vi "RTD_inverse_polynome.vi"(5 "t stop":dbl=95.0, 7 "t start":dbl=5.0, 8 "error in":errorcluster, 11 "channel in":T1={"type"=enum."COMET Tx5xx (ethernet)", "comment"="", "tag"="", "refresh"=5.0, "IP"="192.168.2.34", "port"=502, "VISA"="", "last readout"=timestamp(0 s since 1904-01-01), "TCP ref"=refnum, "VISA sess"="", "idn"="", "press"=0.0, "RH"=0.0, "temp"=0.0, "pres cor"=[], "RH cor"=[], "temp cor"=[], "try left"=0, "failed"=FALSE, "RTD set"=[], "RTD inv"=[], "range"=0.0, "net mode"=enum."MODBUS", "try fail"=enum."Stop trying - return NaN", "timeout [s]"=0.0, "max retries"=0, "sim t [deg]"=0.0, "status"=0} {"status" items=["ok", "retry", "failed"]; "RTD inv" format="%.1f"; "RTD set" format="%.1f"; "temp cor" format="%.1f"; "RH cor" format="%.1f"; "pres cor" format="%.1f"; "refresh" min=0.1 max=1000.0 format="%.2f"}) -> (0 "error out":errorcluster, 3 "channel out":T1={"type"=enum."COMET Tx5xx (ethernet)", "comment"="", "tag"="", "refresh"=5.0, "IP"="192.168.2.34", "port"=502, "VISA"="", "last readout"=timestamp(0 s since 1904-01-01), "TCP ref"=refnum, "VISA sess"="", "idn"="", "press"=0.0, "RH"=0.0, "temp"=0.0, "pres cor"=[], "RH cor"=[], "temp cor"=[], "try left"=0, "failed"=FALSE, "RTD set"=[], "RTD inv"=[], "range"=0.0, "net mode"=enum."MODBUS", "try fail"=enum."Stop trying - return NaN", "timeout [s]"=0.0, "max retries"=0, "sim t [deg]"=0.0, "status"=0} {"status" items=["ok", "retry", "failed"]; "RTD inv" format="%.1f"; "RTD set" format="%.1f"; "temp cor" format="%.1f"; "RH cor" format="%.1f"; "pres cor" format="%.1f"; "refresh" min=0.1 max=1000.0 format="%.2f"})   [LabVIEW 2020]
uses:
  thermo.ctl
  thermo_types.ctl
  Thermometer Fail Action.ctl
panel:
  out "dt set":dbl[](array[numeric])
  out "fit order":i32
  out "XY Graph":cluster{dbl[], dbl[]}(graph)
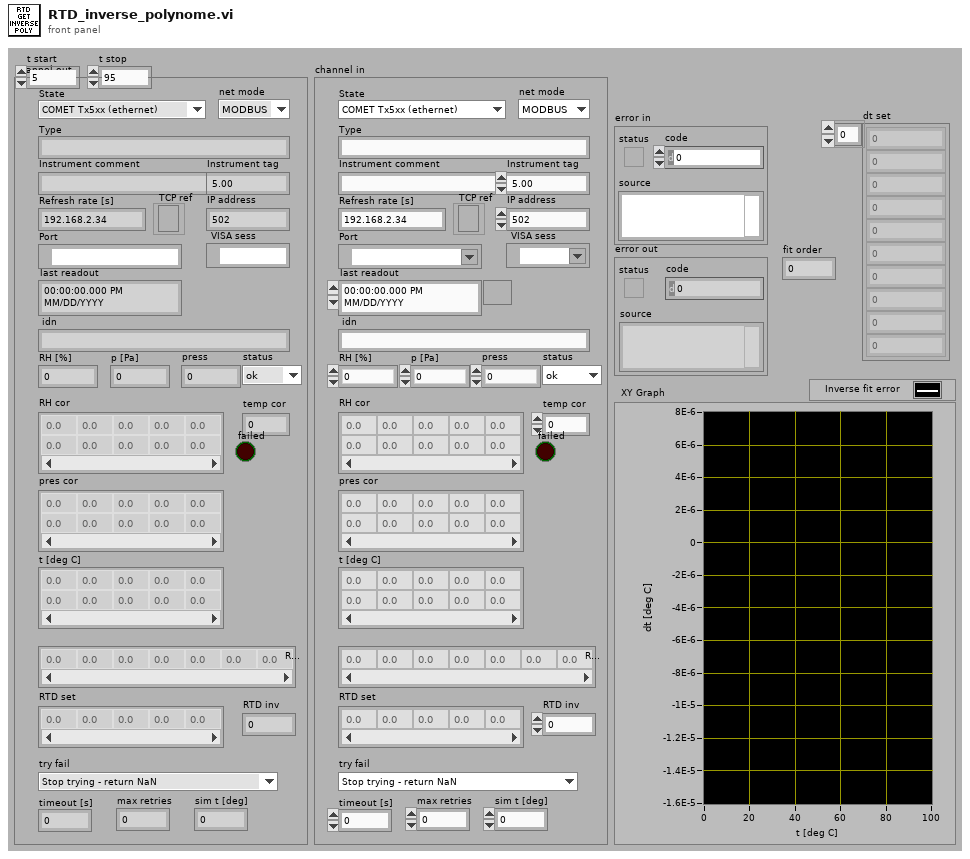
[diagram p1: front panel]
types:
  T1 = typedef "thermo.ctl" = cluster{"type":T2, "comment":string, "tag":string, "refresh":dbl, "IP":string, "port":u16, "VISA":refnum<visa-resource-name>, "last readout":timestamp, "TCP ref":refnum<k5>, "VISA sess":refnum<visa-resource-name>, "idn":string, "press":dbl, "RH":dbl, "temp":dbl, "pres cor":dbl[][], "RH cor":dbl[][], "temp cor":dbl[][], "try left":i32, "failed":bool, "RTD set":dbl[], "RTD inv":dbl[], "range":dbl, "net mode":enum16{"MODBUS", "HTTP"}, "try fail":T3, "timeout [s]":dbl, "max retries":i32, "sim t [deg]":dbl, "status":u16}
  T2 = typedef "thermo_types.ctl" = enum16{"Disabled", "Simulated", "COMET Tx5xx (ethernet)", "Keithley 2002 (GPIB) + RTD", "Agilent 344xx (GPIB) + RTD"}
  T3 = typedef "Thermometer Fail Action.ctl" = enum16{"Stop trying - keep last value", "Stop trying - return NaN", "Generate error - stop sweep"}
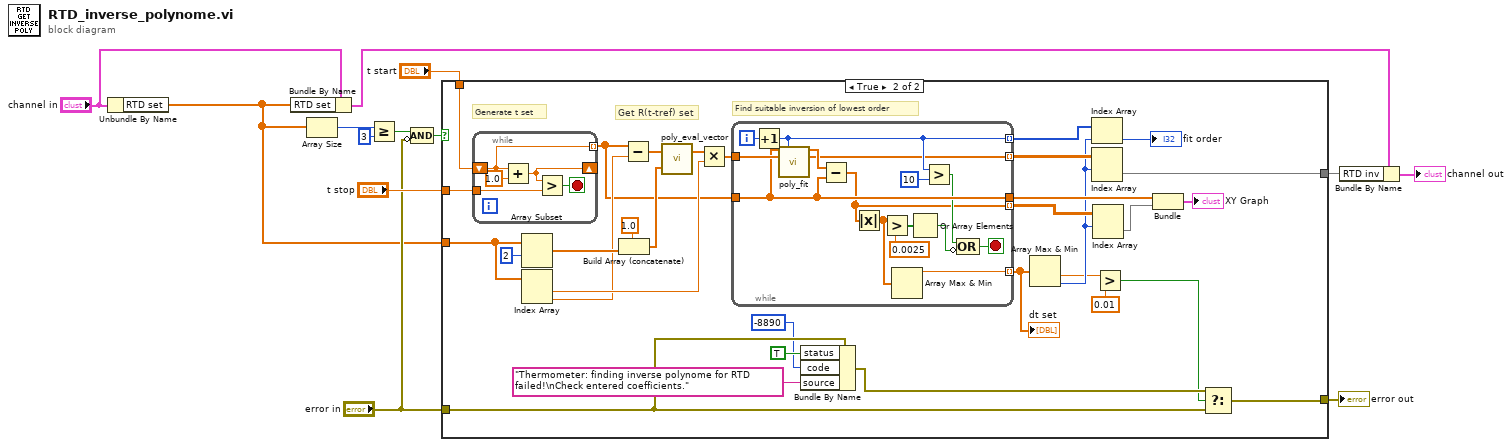
[diagram p0: block diagram]
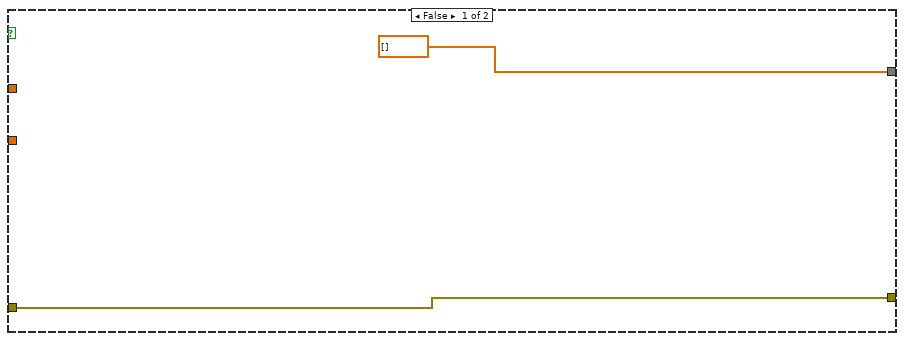
[diagram p2: hidden frame]
diagram:
  n1 = Unbundle By Name("channel in") -> ("RTD set"=w1:dbl[])
  n2 = Bundle By Name(cluster="channel in", "RTD set"=w1) -> (w2:T1)
  n3 = Array Size(array=w1) -> (size(s)=w13:i32)
  n4 = Greater Or Equal?(x=w13, y=3) -> (x >= y?=w9:bool)
  n5 = Compound Arithmetic op=AND(w9, invert "error in") -> (w8:bool)
  n6 = case shown="True" w8 {
    tunnel: "t start" -> [_ w47]
    tunnel: "t stop" -> [_ w46]
    tunnel: w1 -> [_ w39]
    tunnel: "error in" -> [w14 w44]
    tunnel: [dbl[] [] ("Polynomial Coefficients") w25] -> w4
    tunnel: [w14 w45] -> w6
    frame False {
    }
    frame True {
      # "Find suitable inversion of lowest order"
      # "Get R(t-tref) set"
      # "Generate t set"
      n7 = while {
        shift-right: [w64] -> _
        shift-left: w47 -> [w67]
        tunnel: [w67] -> w30 mode=indexing
        tunnel: w46 -> [w63]
        stop <- w65 stop-if-true
        n8 = Add(x=w67, y=1.0) -> (x+y=w64:dbl)
        n9 = Greater?(x=w64, y=w63) -> (0:w65:bool)
      }
      n10 = Array Subset(array=w39, index=2) -> (w38:dbl[])  [unwired: 1 in]
      n11 = Index Array(array=w39) -> (element #1=w36:dbl, element #2=w33:dbl)  [unwired: 2 in]
      n12 = Build Array (concatenate)(1.0 ("y"), w38) -> (w32:dbl[])
      n13 = Subtract(x=w30, y=w33) -> (x-y=w35:dbl[])
      n14 = call "poly_eval_vector.vi"("P(x)"=w32, "A"=w35) -> ("P(A)"=w37:dbl[])  [unwired: 1 in]
      n15 = Multiply(x=w37, y=w36) -> (x*y=w31:dbl[])
      n16 = while {
        tunnel: w31 -> [w60]
        tunnel: w30 -> [w58]
        tunnel: [w58] -> w22
        tunnel: [w52] -> w21 mode=indexing
        tunnel: [w50] -> w27 mode=indexing
        tunnel: [w49] -> w26 mode=indexing
        tunnel: [w48] -> w24 mode=indexing
        i -> [w57]
        stop <- w55 stop-if-true
        n17 = Increment(x=w57) -> (x+1=w52:i32)
        n18 = call "poly_fit.vi"("y"=w58, "order"=w52, "x"=w60) -> ("P(A)"=w59:dbl[], "P(x)"=w49:dbl[])  [unwired: 10 in, 1 out]
        n19 = Subtract(x=w59, y=w58) -> (x-y=w48:dbl[])
        n20 = Absolute Value(x=w48) -> (abs(x)=w51:dbl[])
        n21 = Greater?(x=w51, y=0.0025) -> (0:w61:bool[])
        n22 = Array Max & Min(array=w51) -> (max value=w50:dbl)  [unwired: 3 out]
        n23 = Or Array Elements(Boolean array=w61) -> (logical OR=w53:bool)
        n24 = Greater?(x=w52, y=10) -> (0:w54:bool)
        n25 = Compound Arithmetic op=OR(w54, invert w53) -> (w55:bool)
      }
      "dt set" <- w27
      n26 = Bundle By Name(cluster=w44, "status"=TRUE, "code"=-8890, "source"="Thermometer: finding inverse polynome for RTD failed!\nCheck entered coefficients.") -> (w43:errorcluster)
      n27 = Array Max & Min(array=w27) -> (min value=w18:dbl, min index (indices)=w20:i32)  [unwired: 2 out]
      n28 = Index Array(array=w21, index=w20) -> (element=→"fit order":i32)
      n29 = Index Array(array=w26, index (row)=w20) -> (element=w25:dbl[])  [unwired: 1 in]
      n30 = Index Array(array=w24, index (row)=w20) -> (element=w23:dbl[])  [unwired: 1 in]
      n31 = Greater?(x=w18, y=0.01) -> (0:w17:bool)
      n32 = Bundle(w22, w23) -> (→"XY Graph":cluster{dbl[], dbl[]})  [unwired: 1 in]
      n33 = Select(t=w43, s=w17, f=w44) -> (s? t:f=w45:errorcluster)
    }
  }
  "error out" <- w6
  n34 = Bundle By Name(cluster=w2, "RTD inv"=w4) -> (→"channel out":T1)
